vi "Wait.vi"(0 "value in":refnum<class "Message Enqueuer.lvclass">, 1 "milliseconds to wait":u32) -> (2 "millisecond timer value":u32, 3 "value out":refnum<class "Message Enqueuer.lvclass">)   [LabVIEW 2017]
doc: "Delays the data flow of the wire for a specified period of time."
uses:
  <vilib>/ActorFramework/Message Enqueuer/Message Enqueuer.lvclass
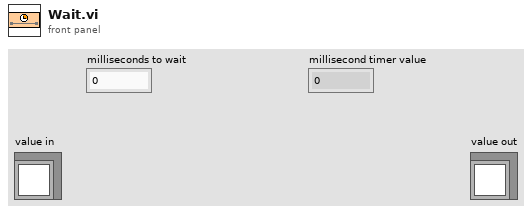
[diagram p1: front panel]
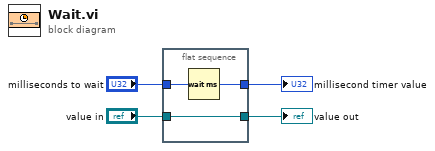
[diagram p0: block diagram]
diagram:
  n1 = flat-sequence {
    tunnel: "milliseconds to wait" -> [w7]
    tunnel: [w6] -> w3
    tunnel: [w5] -> w2
    tunnel: "value in" -> [w5]
    frame #0 {
      n2 = Wait (ms)(milliseconds to wait=w7) -> (millisecond timer value=w6:u32)
    }
  }
  "value out" <- w2
  "millisecond timer value" <- w3
